vi "Clear Sessions.vi"(0 "Session Handle in":T1, 11 "error in (no error)":errorcluster) -> (4 "Session Handle Out":T1, 15 "error out":errorcluster)   [LabVIEW 2015, in "Gas.lvclass"]
uses:
  Gas.lvclass
  Typedefs/Session Handle.ctl
  Gas.lvclass/Gas.ctl
panel:
  out "error out 3":errorcluster
  out "error out 2":errorcluster
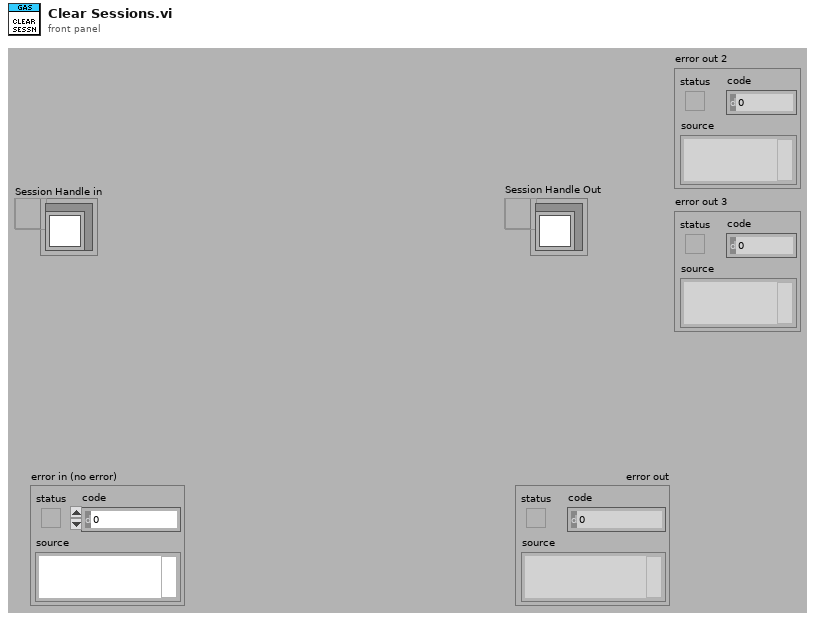
[diagram p1: front panel]
types:
  T1 = typedef "Gas.lvclass/Session Handle.ctl" = refnum<data-value>
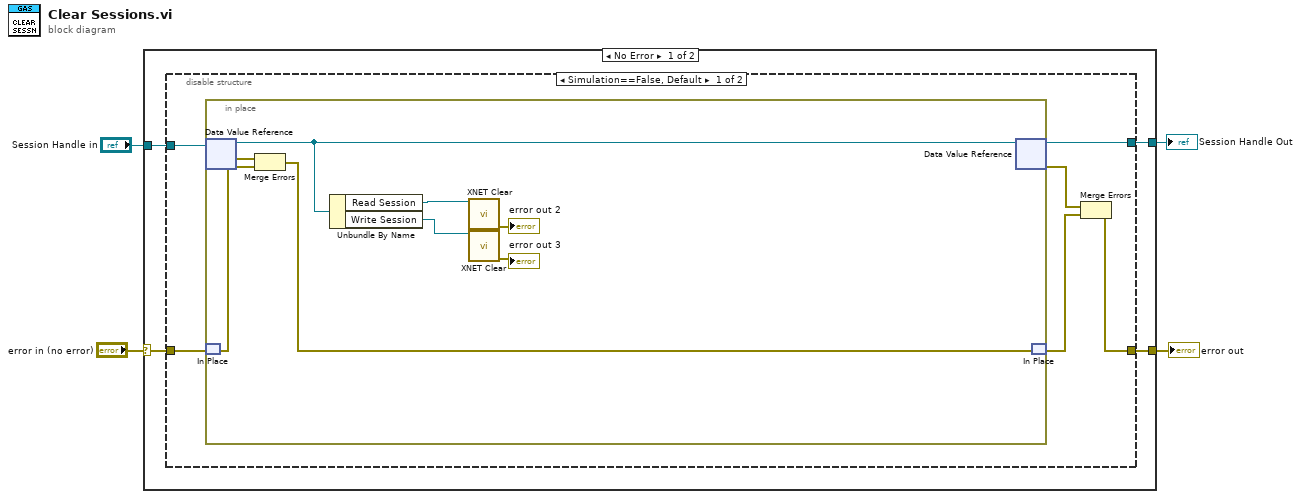
[diagram p0: block diagram]
diagram:
  n1 = case shown="No Error" "error in (no error)" {
    selector: "error in (no error)" -> [w7 w26]
    tunnel: [w8 w26] -> w4
    tunnel: "Session Handle in" -> [w6 w25]
    tunnel: [w5 w25] -> w1
    frame No Error {
      n2 = disable-structure shown="Simulation==False, Default" {
        disable-tunnel: [w12 w23] -> w8
        disable-tunnel: w7 -> [w11 w23]
        disable-tunnel: w6 -> [w10 w24]
        disable-tunnel: [w9 w24] -> w5
        frame condition #0 (active) {
          n3 = in-place {
            n4 = in-place-dvr #1(w10) -> (w20:refnum<class "Gas.lvclass">, w22:errorcluster)
            n5 = in-place-match #2(w11) -> (w21:errorcluster)
            n6 = Merge Errors(w21, w22) -> (w17:errorcluster)
            n7 = Unbundle By Name(w20) -> ("Read Session"=w19:refnum<k21>, "Write Session"=w18:refnum<k21>)
            n8 = call <vilib>:"XNET Clear.vi"("session in"=w19) -> ("error out"=→"error out 2":errorcluster)  [unwired: 14 in]
            n9 = call <vilib>:"XNET Clear.vi"("session in"=w18) -> ("error out"=→"error out 3":errorcluster)  [unwired: 14 in]
            n10 = in-place-dvr #1(w20) -> (w9:T1, w13:errorcluster)
            n11 = in-place-match #2(w17) -> (w14:errorcluster)
          }
          n12 = Merge Errors(w13, w14) -> (w12:errorcluster)
        }
        frame condition #1 {
        }
      }
    }
    frame Error {
    }
  }
  "error out" <- w4
  "Session Handle Out" <- w1
